vi "Update Current Execution Time.vi"(8 "error in":errorcluster, 10 "current execution time (us)":i32, 11 "Execution Unit in":refnum<class "Execution Unit.lvclass">) -> (0 "error out":errorcluster, 3 "Execution Unit out":refnum<class "Execution Unit.lvclass">)   [LabVIEW 2020, in "AIM MIL-STD-1553 Engine.lvlib" / "Implementation.lvlib" / "Execution Unit.lvclass"]
uses:
  Execution Unit.lvclass
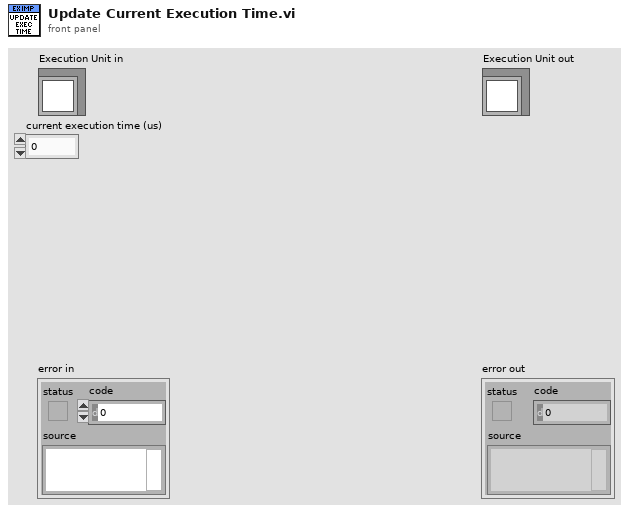
[diagram p1: front panel]
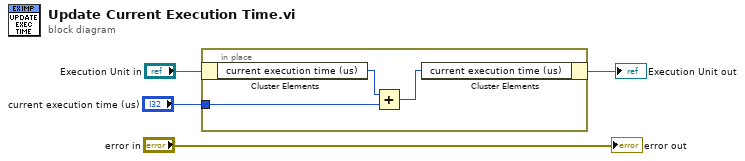
[diagram p0: block diagram]
diagram:
  n1 = in-place {
    in-place-border: "current execution time (us)" -> [w6]
    n2 = in-place-cluster #1("Execution Unit in") -> ("current execution time (us)"=w7:i32)
    n3 = Add(x=w7, y=w6) -> (x+y=w5:i32)
    n4 = in-place-cluster #1("current execution time (us)"=w5) -> (→"Execution Unit out":refnum<class "Execution Unit.lvclass">)
  }
  "error out" <- "error in"
